vi "ResultToList.vi"(7 "CheckDist":bool, 9 "Image In":T1, 10 "ROIList":string[][](array[string]), 11 "ALLResultOut":string[][](array[string])) -> (3 "Result Arr":T2(array[cluster]))   [LabVIEW 2019]
uses:
  <vilib>/vision/Image Controls.llb/IMAQ Image.ctl
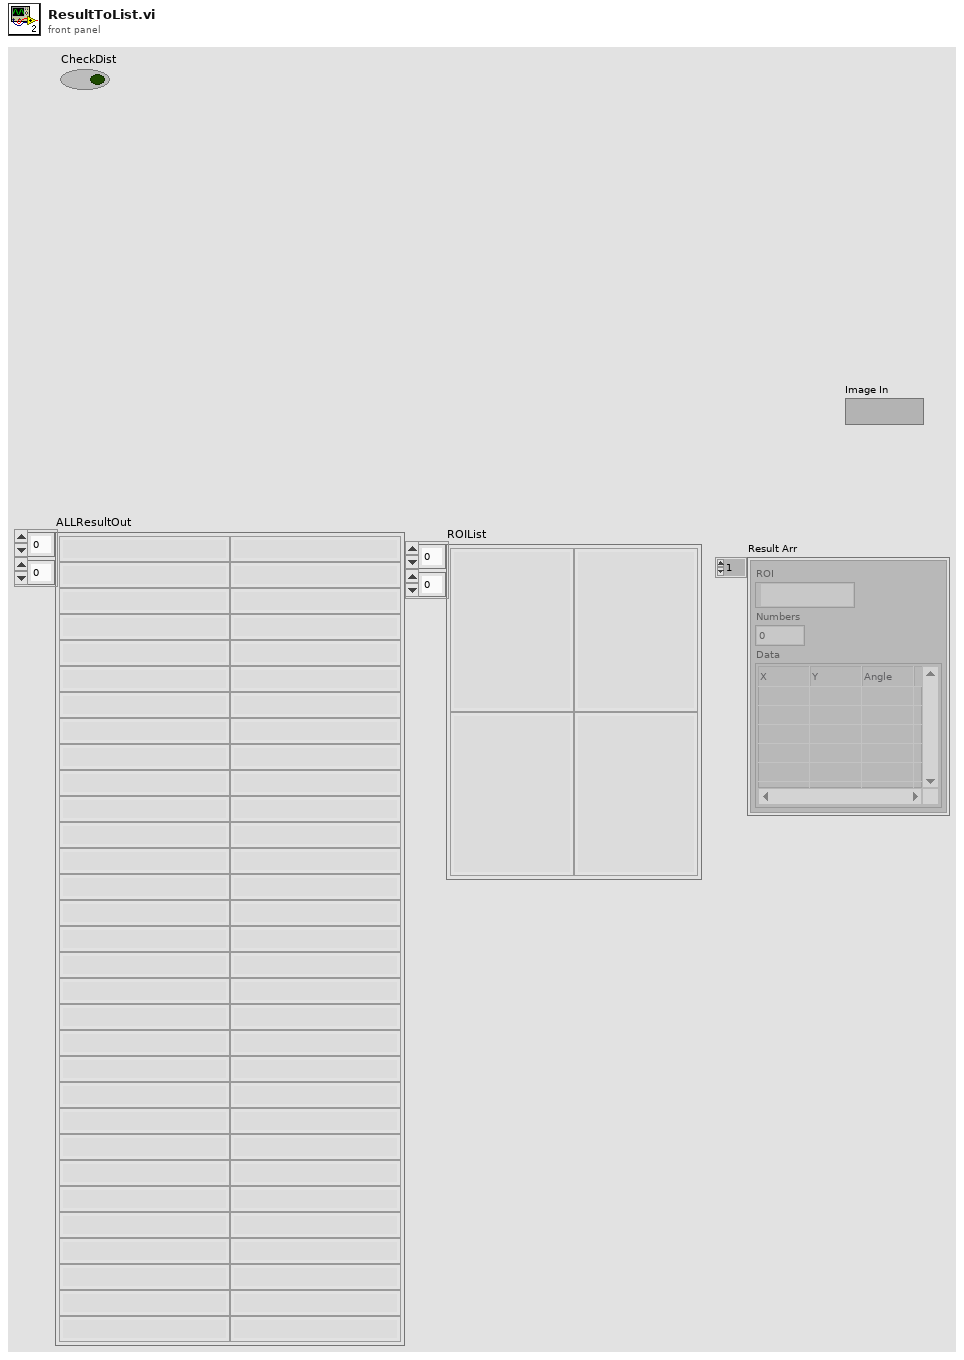
[diagram p1: front panel]
types:
  T1 = typedef "IMAQ Image.ctl" = refnum<image>
  T2 = cluster{"ROI":string, "Numbers":i32, "Data":string[][]}[]
  T3 = enum16{"None", "Image左上", "Image左下", "Image右上", "Image右下"}
  T4 = cluster{"ROI":string, "Numbers":i32, "Data":string[][]}
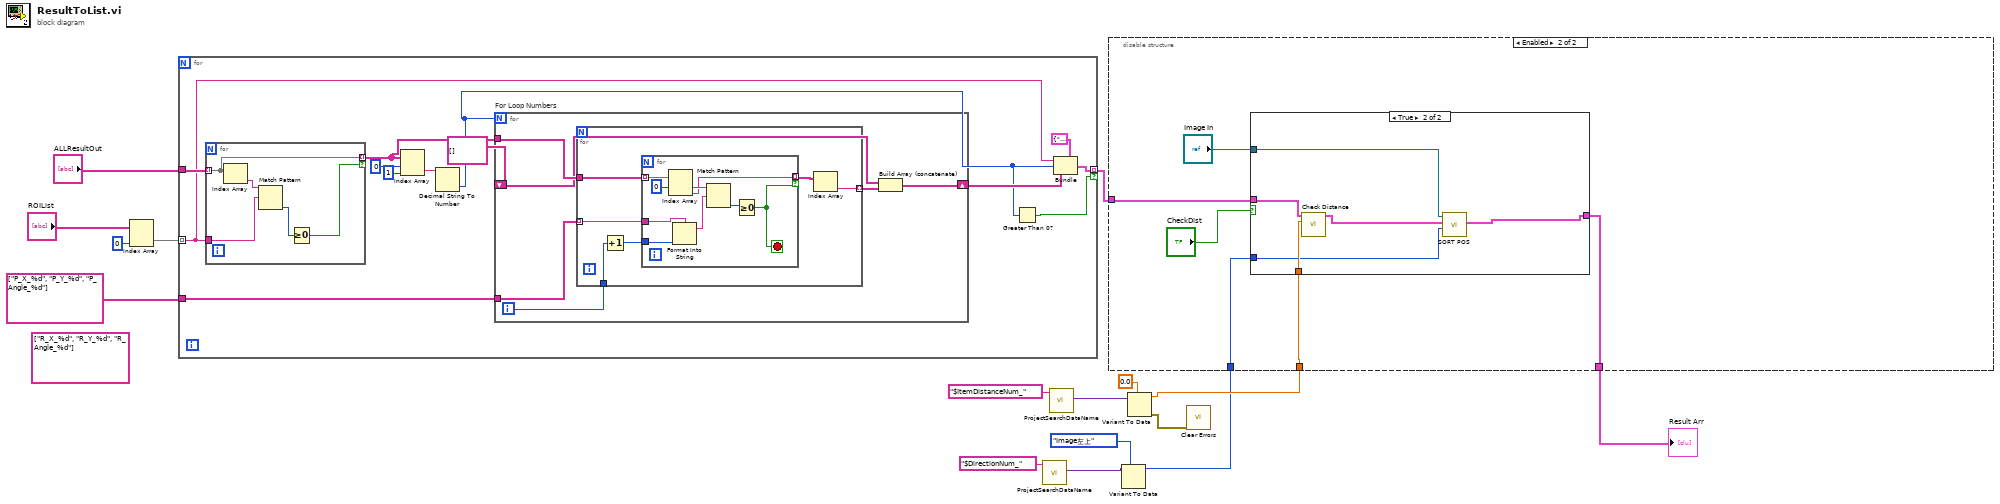
[diagram p0: block diagram]
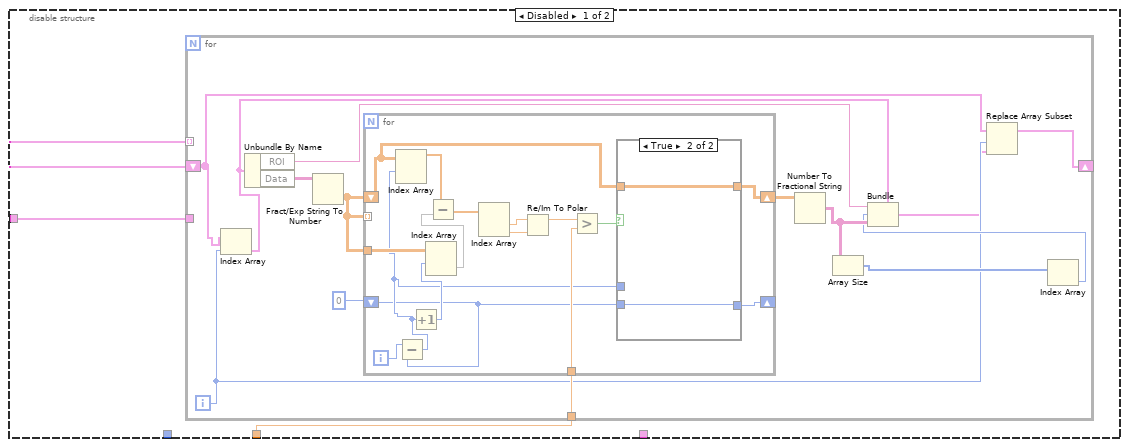
[diagram p2: hidden frame]
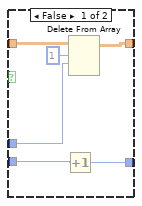
[diagram p3: hidden frame]
diagram:
  (unwired) string[] ["R_X_%d", "R_Y_%d", "R_Angle_%d"]
  n1 = Index Array(array="ROIList", index (col)=0 ("disabled index (col)")) -> (element=w13:string[])  [unwired: 1 in]
  n2 = for {
    tunnel: "ALLResultOut" -> [w29]
    tunnel: w13 -> [w20] mode=indexing
    tunnel: string[] ["P_X_%d", "P_Y_%d", "P_Angle_%d"] -> [w25]
    tunnel: [w21] -> w7 mode=indexing if=w17
    n3 = for {
      tunnel: w20 -> [w54]
      tunnel: w29 -> [w52] mode=indexing
      tunnel: [w52] -> w24 mode=indexing if=w51
      n4 = Index Array(array=w52) -> (element=w55:string)  [unwired: 1 in]
      n5 = Match Pattern(string=w55, regular expression=w54) -> (offset past match=w53:i32)  [unwired: 1 in, 3 out]
      n6 = Greater Or Equal To 0?(x=w53) -> (x >= 0?=w51:bool)
    }
    n7 = Index Array(array=w24, index (row)=0 ("disabled index (row)"), index (col)=1 ("disabled index (col)")) -> (element=w26:string)
    n8 = Decimal String To Number(string=w26) -> (number=w18:i32)  [unwired: 2 in, 1 out]
    n9 = for "For Loop Numbers" {
      N: w18 -> [_]
      tunnel: w25 -> [w35]
      tunnel: w24 -> [w34]
      shift-right: [w31] -> w22
      shift-left: string[][] [] -> [w30]
      i -> [w33]
      n10 = for {
        tunnel: w35 -> [w41] mode=indexing
        tunnel: w34 -> [w40]
        tunnel: w33 -> [w38]
        tunnel: [w36] -> w32 mode=indexing
        n11 = Increment(x=w38) -> (x+1=w39:i32)
        n12 = for {
          tunnel: w41 -> [w49]
          tunnel: w40 -> [w45] mode=indexing
          tunnel: w39 -> [w48]
          tunnel: [w43] -> w37 mode=indexing if=w42
          stop <- w42 stop-if-true
          n13 = Index Array(array=w45, index #1=0 ("index")) -> (element #1=w44:string, element #2=w43:string)  [unwired: 1 in]
          n14 = Format Into String(format string=w49, w48) -> (resulting string=w47:string)  [unwired: 2 in, 1 out]
          n15 = Match Pattern(string=w44, regular expression=w47) -> (offset past match=w46:i32)  [unwired: 1 in, 3 out]
          n16 = Greater Or Equal To 0?(x=w46) -> (x >= 0?=w42:bool)
        }
        n17 = Index Array(array=w37) -> (element=w36:string)  [unwired: 1 in]
      }
      n18 = Build Array (concatenate)(w30, w32) -> (w31:string[][])
    }
    n19 = Greater Than 0?(x=w18) -> (x > 0?=w17:bool)
    n20 = Bundle(cluster=T4 {"ROI"="", "Numbers"=0, "Data"=[]} ("Result"), "ROI"=w20, "Numbers"=w18, "Data"=w22) -> (w21:T4)
  }
  n21 = call "ProjectSearchDataName.vi"("element"="$DirectionNum_") -> ("variant"=w4:variant)  [unwired: 7 in, 3 out]
  n22 = call "ProjectSearchDataName.vi"("element"="$ItemDistanceNum_") -> ("variant"=w10:variant)  [unwired: 7 in, 3 out]
  n23 = Variant To Data(type=T3."Image左上" ("$DirectionNum_"), Variant=w4) -> (data=w1:T3)  [unwired: 1 in, 1 out]
  n24 = Variant To Data(type=0.0, Variant=w10) -> (data=w9:dbl, error out=w5:errorcluster)  [unwired: 1 in]
  n25 = disable-structure shown="Enabled" {
    disable-tunnel: w9 -> [w58 w101]
    disable-tunnel: w7 -> [w56 w102]
    disable-tunnel: [_ w97] -> w6
    disable-tunnel: w1 -> [_ w99]
    frame Disabled {
      n26 = for {
        tunnel: w56 -> [_]
        tunnel: w58 -> [w72]
        shift-right: [w60] -> w57
        shift-left: w56 -> [w63]
        tunnel: w56 -> [_] mode=indexing
        i -> [w62]
        n27 = Index Array(array=w63, index=w62) -> (element=w64:T4)
        n28 = Unbundle By Name(w64) -> ("ROI"=w65:string, "Data"=w71:string[][])
        n29 = Fract/Exp String To Number(string=w71) -> (number=w59:dbl[][])  [unwired: 3 in, 1 out]
        n30 = for {
          tunnel: w59 -> [w84]
          tunnel: w72 -> [w81]
          shift-right: [w78] -> w69
          shift-left: w59 -> [w77]
          shift-right: [w73] -> _
          shift-left: 0 -> [w74]
          tunnel: w59 -> [_] mode=indexing
          i -> [w76]
          n31 = Subtract(x=w76, y=w74) -> (x-y=w75:i32)
          n32 = Index Array(array=w77, index (row)=w75) -> (element=w80:dbl[])  [unwired: 1 in]
          n33 = Increment(x=w75) -> (x+1=w83:i32)
          n34 = Index Array(array=w84, index (row)=w83) -> (element=w82:dbl[])  [unwired: 1 in]
          n35 = Subtract(x=w80, y=w82) -> (x-y=w88:dbl[])
          n36 = Index Array(array=w88) -> (element #1=w86:dbl, element #2=w87:dbl)  [unwired: 2 in]
          n37 = Re/Im To Polar(2:w87, 3:w86) -> (1:w85:dbl)  [unwired: 1 out]
          n38 = Greater?(x=w85, y=w81) -> (0:w79:bool)
          n39 = case shown="True" w79 {
            tunnel: [w93 w96] -> w78
            tunnel: w77 -> [w94 w96]
            tunnel: w75 -> [w91 _]
            tunnel: w74 -> [w90 w95]
            tunnel: [w89 w95] -> w73
            frame False {
              n40 = Increment(x=w90) -> (x+1=w89:i32)
              n41 = Delete From Array(array=w94, length=1, index (row)=w91) -> (array with subset deleted=w93:dbl[][])  [unwired: 1 in, 1 out]
            }
            frame True {
            }
          }
        }
        n42 = Number To Fractional String(number=w69) -> (F-format string=w68:string[][])  [unwired: 3 in]
        n43 = Array Size(array=w68) -> (size(s)=w67:i32[])
        n44 = Index Array(array=w67) -> (element=w66:i32)  [unwired: 1 in]
        n45 = Bundle(cluster=w64, "ROI"=w65, "Numbers"=w66, "Data"=w68) -> (w61:T4)
        n46 = Replace Array Subset(array=w63, new element=w61, index=w62) -> (w60:T2)
      }
    }
    frame Enabled {
      n47 = case shown="True" "CheckDist" {
        tunnel: w102 -> [w103 w109]
        tunnel: [w103 w104] -> w97
        tunnel: w101 -> [_ w108]
        tunnel: w99 -> [_ w107]
        tunnel: "Image In" -> [_ w106]
        frame False {
        }
        frame True {
          n48 = call "Check Distance.vi"("distance"=w108, "Result Arr"=w109) -> ("Array"=w105:T2)  [unwired: 9 in]
          n49 = call "SORT POS.vi"("$DirectionNum_"=w107, "Array in"=w105, "Image In"=w106) -> ("Array out"=w104:T2)  [unwired: 8 in]
        }
      }
    }
  }
  "Result Arr" <- w6
  n50 = call <vilib>:"Clear Errors.vi"("error in (no error)"=w5) -> ()  [unwired: 5 in, 2 out]
